vi "MOdbus TCP Master 反控命令.vi"() -> ()   [LabVIEW 2016]
uses:
  <vilib>/Modbus/subvis/Modbus API/Modbus API.lvclass/Modbus API.ctl
  <vilib>/Modbus/subvis/Transmission Data Unit (ADU)/Transmission Data Unit/Transmission Data Unit.lvclass/Transmission Data Unit.ctl
  <vilib>/Modbus/master/Data Access/Unit ID/Set Unit ID Property.vi
  <vilib>/Modbus/subvis/Transmission Data Unit (ADU)/Transmission Data Unit/Data Access/Unit ID/Write Unit ID.vi
  <vilib>/Modbus/subvis/Modbus API/Read Transmission Data Unit.vi
  <vilib>/Modbus/subvis/Modbus API/Write Transmission Data Unit.vi
  <vilib>/Modbus/master/Modbus Master.lvclass
  F:/Program Files/National Instruments/LabVIEW 2016/vi.lib/Modbus/subvis/Modbus API/Modbus API.lvclass
  <vilib>/Modbus/master/Create Master Instance (Serial).vi
  <vilib>/Modbus/subvis/Transmission Data Unit (ADU)/Transmission Data Unit/Transmission Data Unit.lvclass
panel:
  in  "VISA resource name":refnum<visa-resource-name> caption="VISA资源名称"
  in  "停止":bool
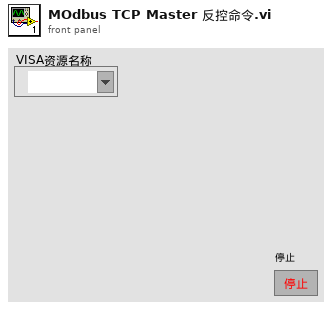
[diagram p1: front panel]
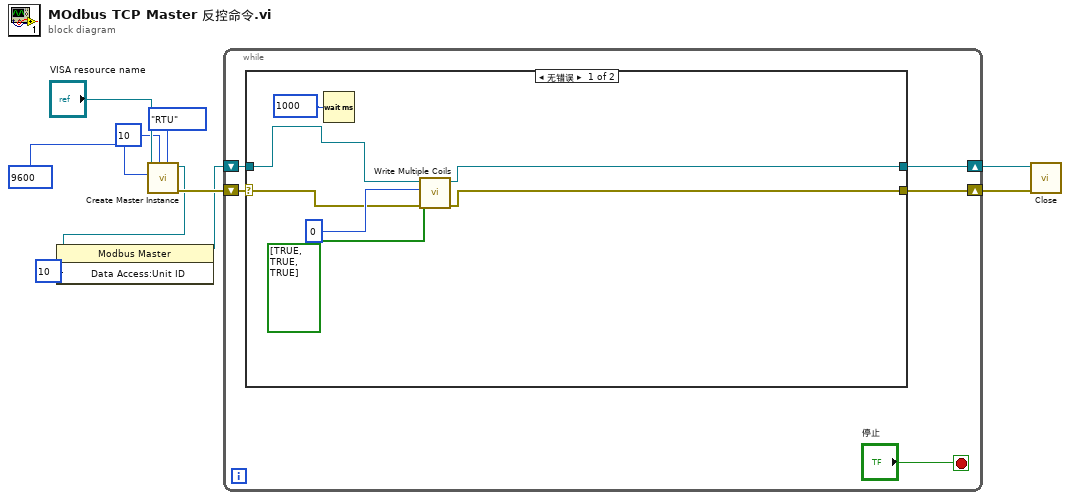
[diagram p0: block diagram]
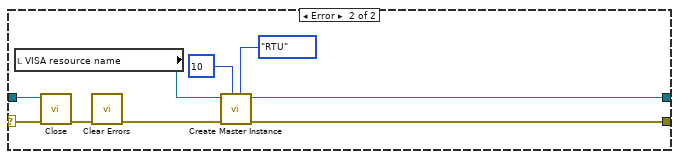
[diagram p2: hidden frame]
diagram:
  n1 = call-poly <vilib>:"Create Master Instance.vi"("serial type"=enum16{"RTU", "ASCII"}."RTU", "unit ID"=u8 10, "baud rate (9600)"=u32 9600, "VISA resource name"="VISA resource name") -> ("error out"=w10:errorcluster, "serial master instance"=w1:refnum<class "Modbus Master.lvclass">)  [unwired: 6 in]
  n2 = property class="Modbus Master"(reference=w1, "Data Access:Unit ID"=u8 10 ("Unit ID")) -> (reference out=w7:refnum<class "Modbus Master.lvclass">)  [unwired: 1 in, 1 out]
  n3 = while {
    shift-right: [w13] -> w8
    shift-left: w10 -> [w12]
    shift-right: [w14] -> w9
    shift-left: w7 -> [w15]
    stop <- "停止" stop-if-true
    n4 = case shown="无错误" w12 {
      selector: w12 -> [w18 w31]
      tunnel: w15 -> [w21 w30]
      tunnel: [w17 w26] -> w14
      tunnel: [w16 w27] -> w13
      frame No Error {
        n5 = Wait (ms)(milliseconds to wait=u32 1000 ("等待时间（毫秒）")) -> ()  [unwired: 1 out]
        n6 = call-dynamic "Write Multiple Coils.vi"("error in (no error)"=w18, "coil values"=bool[] [TRUE, TRUE, TRUE], "starting address"=u16 0, "Modbus master in"=w21) -> ("error out"=w16:errorcluster, "Modbus master out"=w17:refnum<class "Modbus Master.lvclass">)  [unwired: 6 in]
      }
      frame Error {
        n7 = local read "VISA resource name"() -> (w23:refnum<visa-resource-name>)
        n8 = call-dynamic "Close.vi"("error in (no error)"=w31, "Modbus master in"=w30) -> ("error out"=w29:errorcluster)  [unwired: 9 in]
        n9 = call <vilib>:"Clear Errors.vi"("error in (no error)"=w29) -> ("error out"=w28:errorcluster)  [unwired: 5 in, 1 out]
        n10 = call-poly <vilib>:"Create Master Instance.vi"("serial type"=enum16{"RTU", "ASCII"}."RTU", "unit ID"=u8 10, "error in (no error)"=w28, "VISA resource name"=w23) -> ("error out"=w27:errorcluster, "serial master instance"=w26:refnum<class "Modbus Master.lvclass">)  [unwired: 6 in]
      }
    }
  }
  n11 = call-dynamic "Close.vi"("error in (no error)"=w8, "Modbus master in"=w9) -> ()  [unwired: 9 in, 1 out]
